vi "Delete directory.vi"(6 "Paths to exclude":string[](array[string]), 8 "error in (no error)":errorcluster, 9 "Contents only? (true)":bool=TRUE, 10 "Directory":string, 11 "File Transfer Behavior in":refnum<class "File Transfer Behavior.lvclass">) -> (0 "error out":errorcluster, 3 "File Transfer Behavior out":refnum<class "File Transfer Behavior.lvclass">)   [LabVIEW 2015, in "RT Management.lvlib" / "File Transfer Behavior.lvclass"]
doc: "Deletes a directory and all contents, both directories and files. If \"Contents only?\" is true (default), then the only the contents of the directory are deleted and the directory is left. If false, the directory itself and all contents are deleted.\n\n\"Paths to exclude\" are paths that you do not want deleted. If a directory is included here, all of its contents, including all sub-directories and files, will be excluded from the delete.\n\nThe recommended file path format for \"Remote path\" is \"/directory1/directory2\" or \"/directory/filename.extension\". However, the VI will accept other formats and transform the path appropriately in most cases. Use the \"Strip path.vi\" and \"Build path.vi\" VIs to help with handling remote path strings."
uses:
  File Transfer Behavior.lvclass
  Fix path [scalar].vi
  <vilib>/Utility/error.llb/Trim Whitespace.vi
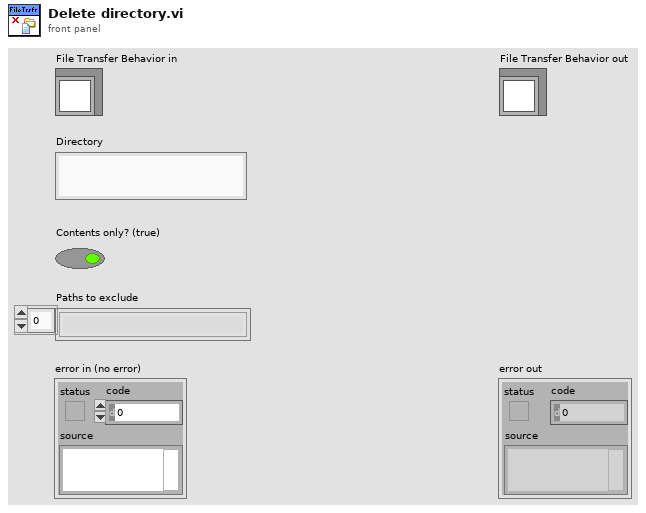
[diagram p1: front panel]
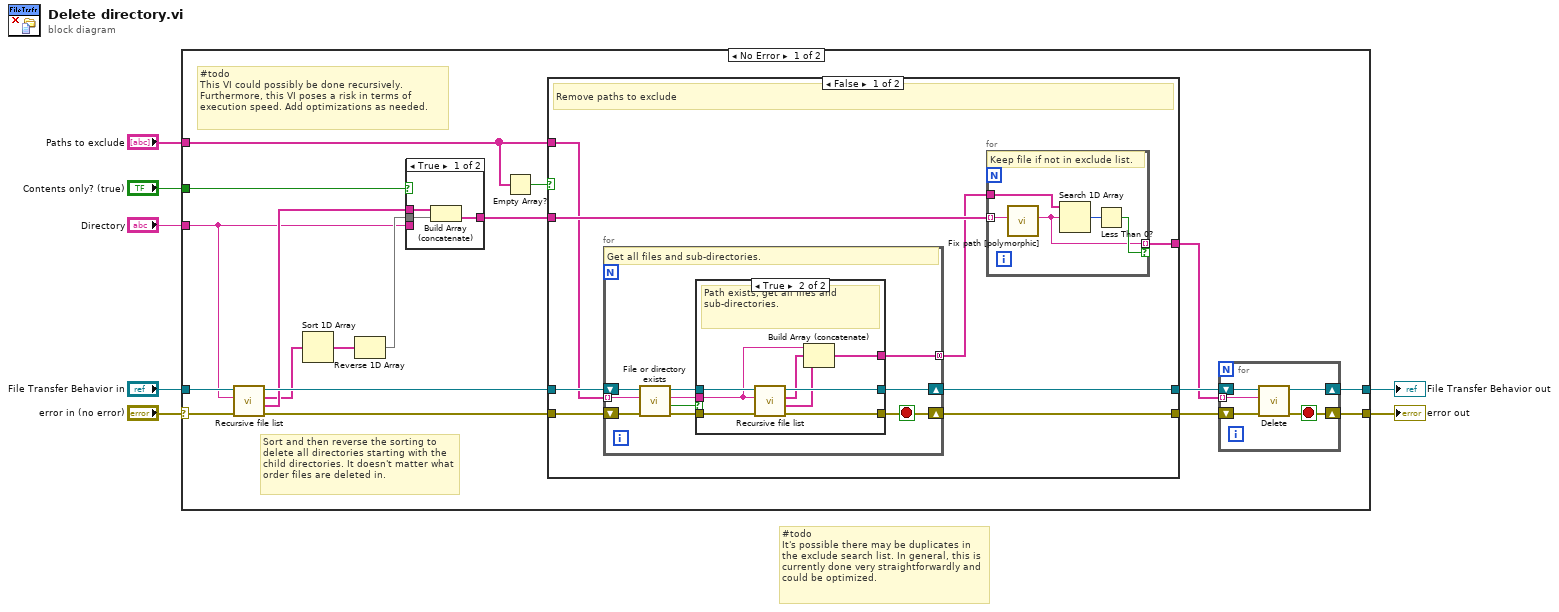
[diagram p0: block diagram]
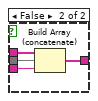
[diagram p4: hidden frame]
diagram:
  # "#todo\nIt's possible there may be duplicates in the exclude search list. In general, this is currently done very straightforwardly and could be optimized."
  n1 = case shown="No Error" "error in (no error)" {
    selector: "error in (no error)" -> [w23 w75]
    tunnel: [w20 w75] -> w6
    tunnel: [w19 w74] -> w4
    tunnel: "File Transfer Behavior in" -> [w22 w74]
    tunnel: "Directory" -> [w15 _]
    tunnel: "Contents only? (true)" -> [w14 _]
    tunnel: "Paths to exclude" -> [w10 _]
    frame No Error {
      # "#todo\nThis VI could possibly be done recursively. Furthermore, this VI poses a risk in terms of execution speed. Add optimizations as needed."
      # "Sort and then reverse the sorting to delete all directories starting with the child directories. It doesn't matter what order files are deleted in."
      n2 = call-dynamic "Recursive file list.vi"("error in (no error)"=w23, "Path"=w15, "File Transfer Behavior in"=w22) -> ("error out"=w9:errorcluster, "Files"=w18:string[], "Directories"=w16:string[], "File Transfer Behavior out"=w24:refnum<class "File Transfer Behavior.lvclass">)  [unwired: 5 in]
      n3 = Sort 1D Array(array=w16) -> (sorted array=w21:string[])
      n4 = Reverse 1D Array(array=w21) -> (reversed array=w17:string[])
      n5 = case shown="True" w14 {
        tunnel: w18 -> [w64 w68]
        tunnel: w17 -> [w63 w67]
        tunnel: [w62 w66] -> w13
        tunnel: w15 -> [_ w65]
        frame True {
          n6 = Build Array (concatenate)(w64, w63) -> (w62:string[])
        }
        frame False {
          n7 = Build Array (concatenate)(w68, w67, w65) -> (w66:string[])
        }
      }
      n8 = Empty Array?(array=w10) -> (empty?=w11:bool)
      n9 = case shown="False" w11 {
        tunnel: w13 -> [w33 w61]
        tunnel: [w32 w61] -> w12
        tunnel: w10 -> [w27 _]
        tunnel: w9 -> [w31 w59]
        tunnel: w24 -> [w28 w60]
        tunnel: [w30 w59] -> w8
        tunnel: [w29 w60] -> w25
        frame False {
          # "Remove paths to exclude"
          n10 = for {
            shift-right: [w43] -> w29
            shift-left: w28 -> [w39]
            shift-right: [w41] -> w30
            shift-left: w31 -> [w40]
            tunnel: w27 -> [w38] mode=indexing
            tunnel: [w42] -> w26 mode=concatenating
            stop <- w41 stop-if-true
            # "Get all files and sub-directories."
            n11 = call-dynamic "File or directory exists.vi"("error in (no error)"=w40, "Path"=w38, "File Transfer Behavior in"=w39) -> ("error out"=w37:errorcluster, "Exists?"=w34:bool, "Path out (dup)"=w35:string, "File Transfer Behavior out"=w36:refnum<class "File Transfer Behavior.lvclass">)  [unwired: 4 in, 1 out]
            n12 = case shown="True" w34 {
              tunnel: [w44 w53] -> w43
              tunnel: [_ w50] -> w42
              tunnel: [w45 w49] -> w41
              tunnel: w37 -> [w45 w48]
              tunnel: w36 -> [w44 w47]
              tunnel: w35 -> [_ w46]
              frame False {
                # "If a path to exclude doesn't exist, we don't need to do anything."
              }
              frame True {
                # "Path exists, get all files and sub-directories."
                n13 = call-dynamic "Recursive file list.vi"("error in (no error)"=w48, "Path"=w46, "File Transfer Behavior in"=w47) -> ("error out"=w49:errorcluster, "Files"=w51:string[], "Directories"=w52:string[], "File Transfer Behavior out"=w53:refnum<class "File Transfer Behavior.lvclass">)  [unwired: 5 in]
                n14 = Build Array (concatenate)(w46, w52, w51) -> (w50:string[])
              }
            }
          }
          n15 = for {
            tunnel: w33 -> [w55] mode=indexing
            tunnel: w26 -> [w58]
            tunnel: [w54] -> w32 mode=indexing if=w56
            # "Keep file if not in exclude list."
            n16 = call-poly "Fix path [polymorphic].vi"("Path in"=w55) -> ("Path out"=w54:string)  [unwired: 8 in, 2 out]
            n17 = Search 1D Array(1D array=w58, element=w54) -> (index of element=w57:i32)  [unwired: 1 in]
            n18 = Less Than 0?(x=w57) -> (x < 0?=w56:bool)
          }
        }
        frame True {
        }
      }
      n19 = for {
        tunnel: w12 -> [w70] mode=indexing
        shift-right: [w69] -> w20
        shift-left: w8 -> [w73]
        shift-right: [w72] -> w19
        shift-left: w25 -> [w71]
        stop <- w69 stop-if-true
        n20 = call-dynamic "Delete.vi"("error in (no error)"=w73, "Path"=w70, "File Transfer Behavior in"=w71) -> ("error out"=w69:errorcluster, "File Transfer Behavior out"=w72:refnum<class "File Transfer Behavior.lvclass">)  [unwired: 7 in]
      }
    }
    frame Error {
    }
  }
  "error out" <- w6
  "File Transfer Behavior out" <- w4
